vi "Scan_BU.vi"(7 "current_mode":u8[](array[numeric])=[0, 0, 0, 0, 0, 0, 0, 0, 0, 0, 0], 8 "ESP32 error":errorcluster, 9 "ESP32 ref":refnum<visa-resource-name>, 10 "DMM error":errorcluster, 11 "DMM ref":refnum<visa-resource-name>) -> (0 "ESP32 error":errorcluster, 1 "ESP32 ref":refnum<visa-resource-name>, 2 "DMM error":errorcluster, 3 "DMM ref":refnum<visa-resource-name>, 4 "Time out count":i32, 5 "Measurements":dbl[](array[numeric]), 6 "Timout?":bool)   [LabVIEW 2023]
uses:
  <instrlib>/Agilent 3446X Series/Agilent 3446X Series.lvlib
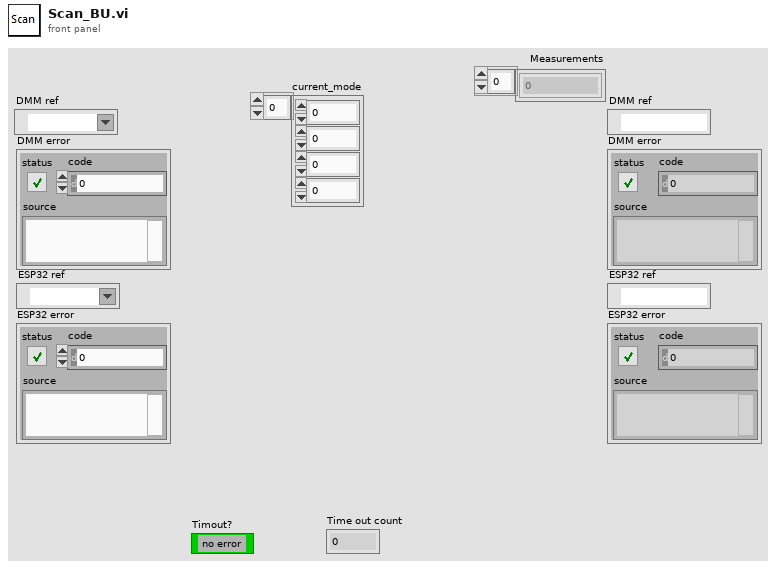
[diagram p1: front panel]
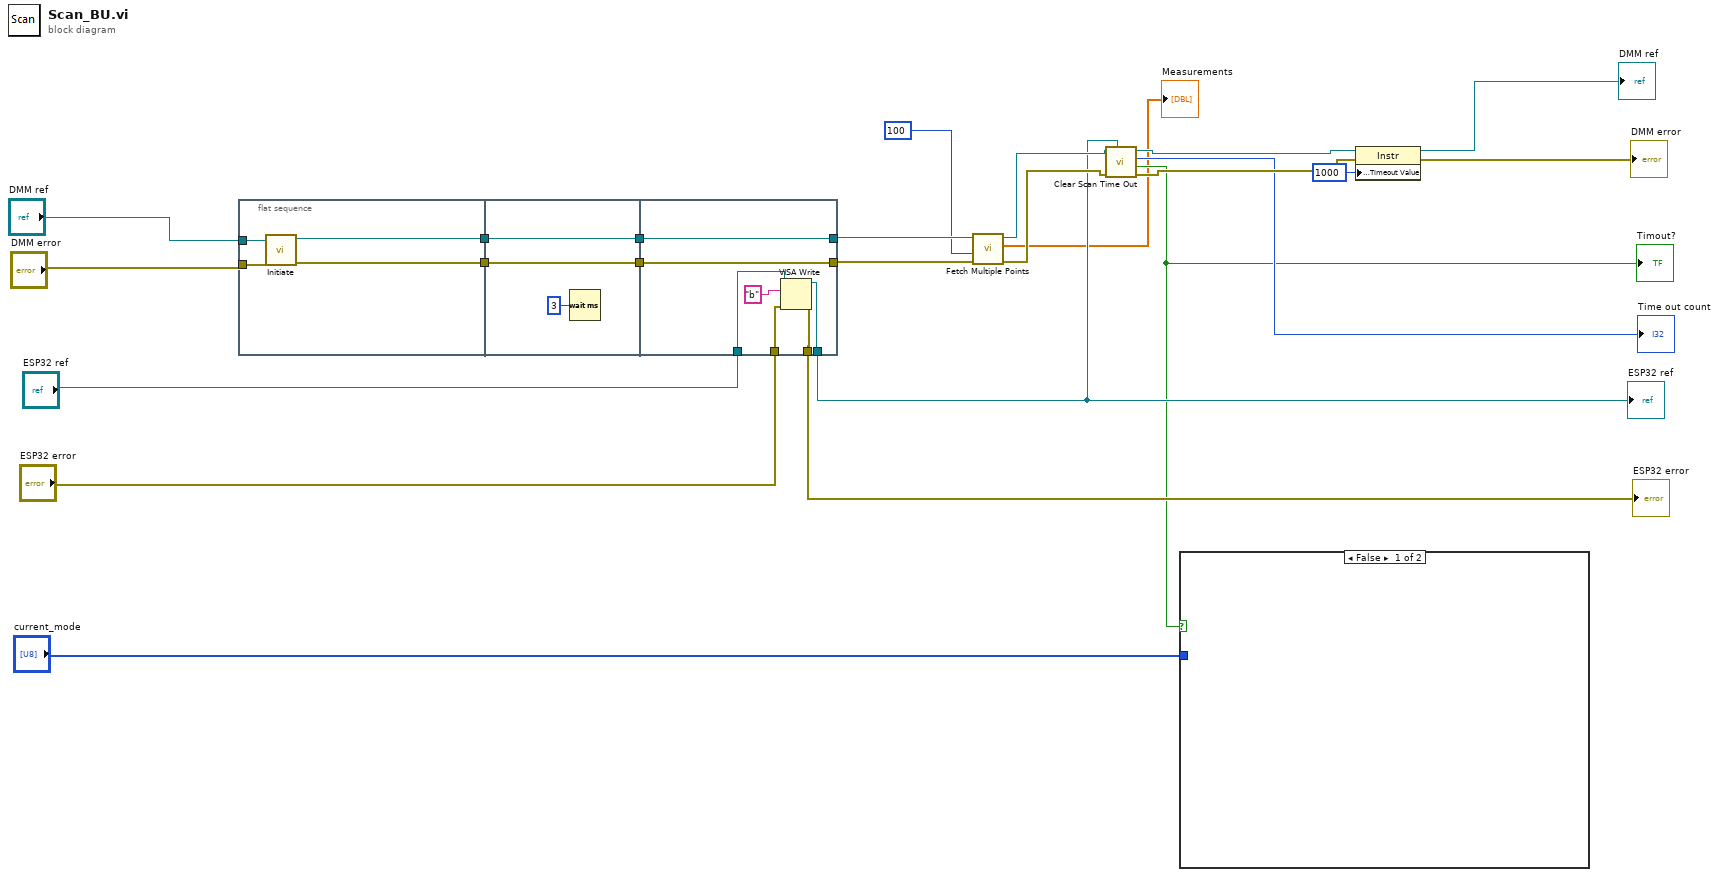
[diagram p0: block diagram]
diagram:
  n1 = flat-sequence {
    tunnel: [w28] -> w24
    tunnel: [w27] -> w23
    tunnel: "DMM ref" -> [w26]
    tunnel: "DMM error" -> [w25]
    tunnel: w24 -> [w31]
    tunnel: [w31] -> w22
    tunnel: w23 -> [w30]
    tunnel: [w30] -> w21
    tunnel: w22 -> [w38]
    tunnel: w21 -> [w37]
    tunnel: "ESP32 ref" -> [w36]
    tunnel: "ESP32 error" -> [w35]
    tunnel: [w34] -> w5
    tunnel: [w33] -> w6
    tunnel: [w38] -> w20
    tunnel: [w37] -> w19
    frame #0 {
      n2 = call <instrlib>:"Initiate.vi"("error in (no error)"=w25, "VISA resource name"=w26) -> ("error out"=w28:errorcluster, "VISA resource name out"=w27:refnum<visa-resource-name>)  [unwired: 8 in]
    }
    frame #1 {
      n3 = Wait (ms)(milliseconds to wait=u32 3) -> ()  [unwired: 1 out]
    }
    frame #2 {
      n4 = VISA Write(VISA resource name=w36, write buffer="b" ("data in"), error in (no error)=w35) -> (VISA resource name out=w34:refnum<visa-resource-name>, error out=w33:errorcluster)  [unwired: 1 out]
    }
  }
  n5 = call <instrlib>:"Fetch Multiple Points.vi"("error in (no error)"=w20, "Timeout (10000 ms)"=100, "VISA resource name"=w19) -> ("error out"=w15:errorcluster, "Measurements"=→"Measurements":dbl[], "VISA resource name out"=w16:refnum<visa-resource-name>)  [unwired: 1 in, 5 out]
  n6 = call "Clear Scan Time Out.vi"("ESP32 ref"=w5, "error in (no error)"=w15, "VISA Refnum in"=w16) -> ("error out"=w13:errorcluster, "error?"=w3:bool, "Time out count"=→"Time out count":i32, "VISA Refnum out"=w14:refnum<visa-resource-name>)  [unwired: 5 in]
  "Timout?" <- w3
  n7 = case shown="False" w3 {
    tunnel: "current_mode" -> [_ _]
    frame False {
    }
    frame True {
    }
  }
  n8 = property class="Instr"(reference=w14, error in=w13, "General Settings:Timeout Value"=u32 1000) -> (reference out=→"DMM ref":refnum<visa-resource-name>, error out=→"DMM error":errorcluster)
  "ESP32 ref" <- w5
  "ESP32 error" <- w6
